vi "pico retract.vi"(8 "error in":errorcluster, 11 "Coarse Approach":refnum<class "Coarse Approach.lvclass">) -> (0 "error out":errorcluster, 2 "Position":i32, 3 "Coarse Approach":refnum<class "Coarse Approach.lvclass">)   [LabVIEW 2020, in "Coarse Approach.lvclass"]
uses:
  Coarse Approach.lvclass
  Coarse Approach.lvclass/Coarse Approach.ctl
  Picomotor/Picomotor.lvclass
panel:
  in  "Destination (steps)":i16=10000
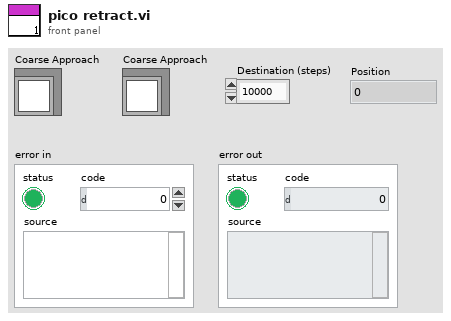
[diagram p1: front panel]
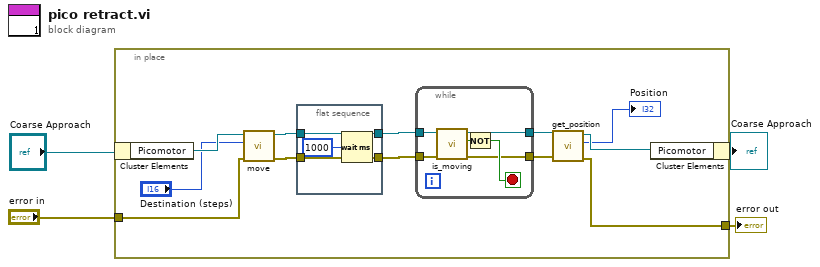
[diagram p0: block diagram]
diagram:
  n1 = in-place {
    in-place-border: "error in" -> [w15]
    in-place-border: [w11] -> w1
    n2 = in-place-cluster #1("Coarse Approach") -> ("Picomotor"=w16:refnum<class "Picomotor.lvclass">)
    n3 = call-dynamic "move.vi"("error in"=w15, "Destination (steps)"="Destination (steps)", "Picomotor in"=w16) -> ("error out"=w7:errorcluster, "Picomotor out"=w8:refnum<class "Picomotor.lvclass">)  [unwired: 7 in]
    n4 = flat-sequence {
      tunnel: w8 -> [w18]
      tunnel: w7 -> [w17]
      tunnel: [w18] -> w6
      tunnel: [w17] -> w5
      frame #0 {
        n5 = Wait (ms)(milliseconds to wait=u32 1000) -> ()  [unwired: 1 out]
      }
    }
    n6 = while {
      tunnel: w6 -> [w23]
      tunnel: w5 -> [w22]
      tunnel: [w21] -> w13
      tunnel: [w20] -> w12
      stop <- w24 stop-if-true
      n7 = call-dynamic "is_moving.vi"("error in (no error)"=w22, "Picomotor in"=w23) -> ("error out"=w20:errorcluster, "Is moving?"=w25:bool, "Picomotor out"=w21:refnum<class "Picomotor.lvclass">)  [unwired: 7 in]
      n8 = Not(x=w25) -> (.not. x?=w24:bool)
    }
    n9 = call-dynamic "get_position.vi"("error in"=w12, "Picomotor in"=w13) -> ("error out"=w11:errorcluster, "Position"=→"Position":i32, "Picomotor out"=w10:refnum<class "Picomotor.lvclass">)  [unwired: 7 in]
    n10 = in-place-cluster #1("Picomotor"=w10) -> (→"Coarse Approach":refnum<class "Coarse Approach.lvclass">)
  }
  "error out" <- w1
